vi "LauncheListner.vi"(8 "error in (no error)":errorcluster, 11 "TCP_Server in":refnum<class "TCP_Server.lvclass">) -> (0 "error out":errorcluster, 3 "TCP_Server out":refnum<class "TCP_Server.lvclass">)   [LabVIEW 2023, in "TCP_Server.lvlib" / "TCP_Server.lvclass"]
uses:
  TCP_Server.lvclass
  C:/Program Files (x86)/National Instruments/LabVIEW 2023/vi.lib/ActorFramework/Actor/Actor.lvclass
  TCP_Listener/TCP_Listener/TCP_Listener.lvclass
  TCP_Server.lvclass/TCP_Server.ctl
  TCP_Listener/TCP_Listener Messages/Write Error Logger's Enqueuer Msg/Write Error Logger's Enqueuer Msg.lvclass/Write Error Logger's Enqueuer Msg.ctl
  <vilib>/ActorFramework/Message Enqueuer/Message Enqueuer.lvclass/Message Enqueuer.ctl
  <vilib>/ActorFramework/Message Enqueuer/Enqueue.vi
  TCP_Listener/TCP_Listener Messages/Write Error Logger's Enqueuer Msg/Write Error Logger's Enqueuer Msg.lvclass
  C:/Program Files (x86)/National Instruments/LabVIEW 2023/vi.lib/ActorFramework/Message/Message.lvclass
  <vilib>/ActorFramework/Message Priority Queue/Priority Enqueue.vi
  <vilib>/ActorFramework/Actor/Actor.lvclass
  C:/Source/LabVIEW/TCP_server/TCP_Listener/TCP_Listener/TCP_Listener.lvclass
  C:/Source/LabVIEW/TCP_server/TCP_Server/TCP_Server/TCP_Server.lvclass
  C:/Source/LabVIEW/TCP_server/TCP_Client_Window/TCP_ClientWindow_Controller/TCP_ClientWindow_Controller.lvclass
  C:/Source/LabVIEW/TCP_server/TCP_Listener/Connections Controller/Connections Controller.lvclass
  C:/Source/LabVIEW/TCP_server/TCP_Server_Connection_Handler/TCP_Connections_Controller/TCP_Connections_Controller.lvclass
  C:/Source/LabVIEW/TCP_server/SimpleErrorLogger/ApplicationWithErrorLogger/ApplicationWithErrorLogger.lvclass
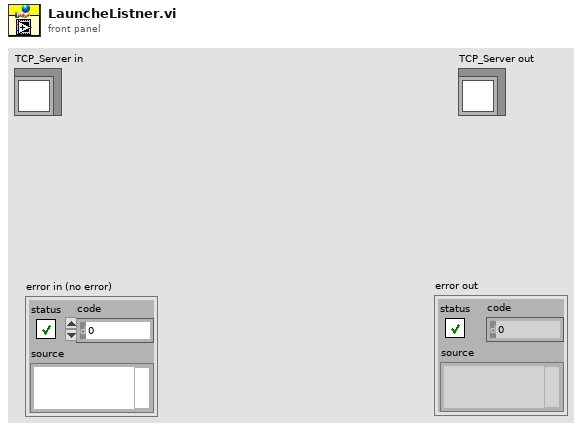
[diagram p1: front panel]
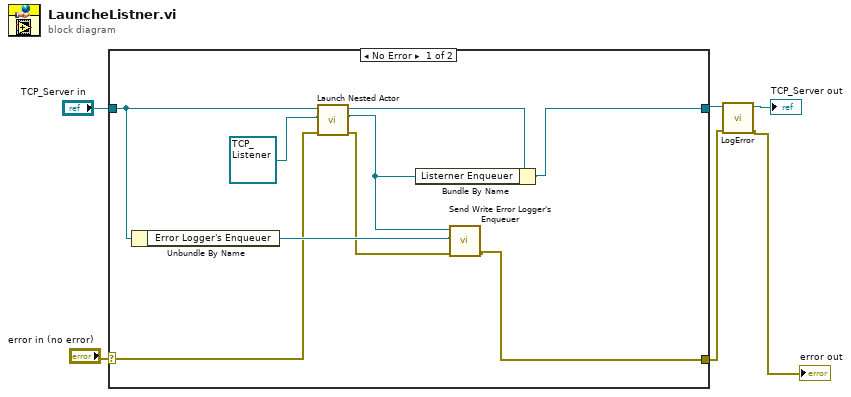
[diagram p0: block diagram]
diagram:
  n1 = case shown="No Error" "error in (no error)" {
    selector: "error in (no error)" -> [w9 w17]
    tunnel: [w7 w17] -> w2
    tunnel: [w13 w16] -> w4
    tunnel: "TCP_Server in" -> [w11 w16]
    frame No Error {
      n2 = Unbundle By Name(w11) -> ("Error Logger's Enqueuer"=w10:refnum<class "Message Enqueuer.lvclass">)
      n3 = call <vilib>:"Launch Nested Actor.vi"("error in (no error)"=w9, "Nested Actor"=refnum<class "TCP_Listener.lvclass"> refnum ("TCP_Listener.lvlib:TCP_Listener.lvclass"), "Caller Actor in"=w11) -> ("error out"=w8:errorcluster, "Nested Actor's Enqueuer"=w12:refnum<class "Message Enqueuer.lvclass">, "Caller Actor out"=w14:refnum<class "TCP_Server.lvclass">)  [unwired: 6 in]
      n4 = Bundle By Name(cluster=w14, "Listerner Enqueuer"=w12) -> (w13:refnum<class "TCP_Server.lvclass">)
      n5 = call "Send Write Error Logger's Enqueuer.vi"("error in (no error)"=w8, "Actor Framework:Message Enqueuer"=w10, "Message Enqueuer"=w12) -> ("error out"=w7:errorcluster)  [unwired: 7 in, 1 out]
    }
    frame Error {
    }
  }
  n6 = call "LogError.vi"("error in (no error)"=w2, "TCP_Server in"=w4) -> ("error out"=→"error out":errorcluster, "TCP_Server out"=→"TCP_Server out":refnum<class "TCP_Server.lvclass">)  [unwired: 8 in]
